vi "Find Config File.vi"(8 "error in (no error)":errorcluster, 11 "Library Path":path) -> (0 "error out":errorcluster, 2 "Config File Exists?":bool, 3 "Ini File Path":path)   [LabVIEW 2019, in "PPL INI Parsing.lvlib"]
uses:
  PPL INI Parsing.lvlib
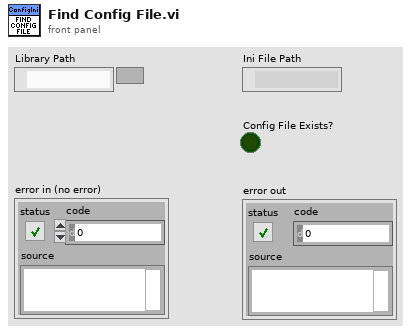
[diagram p1: front panel]
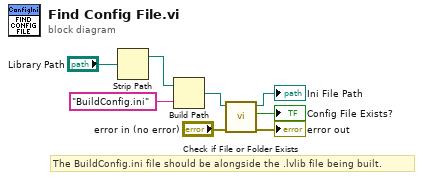
[diagram p0: block diagram]
diagram:
  # "The BuildConfig.ini file should be alongside the .lvlib file being built."
  n1 = Strip Path(path="Library Path") -> (stripped path=w2:path)  [unwired: 1 out]
  n2 = Build Path(base path=w2, name or relative path="BuildConfig.ini") -> (appended path=w8:path)
  n3 = call <vilib>:"Check if File or Folder Exists.vi"("error in (no error)"="error in (no error)", "path"=w8) -> ("error out"=→"error out":errorcluster, "file or folder exists?"=→"Config File Exists?":bool, "dup path"=→"Ini File Path":path)  [unwired: 7 in]
